vi "Register Check Running.vi"(8 "error in (no error)":errorcluster, 11 "Check Running (F)":bool) -> (0 "error out":errorcluster, 3 "Running?":bool)   [LabVIEW 2013, in "Caraya.lvlib" / "Basic Test Manager.lvclass"]
uses:
  Basic Test Manager.lvclass
  <userlib>/_OpenG.lib/array/array.llb/Conditional Auto-Indexing Tunnel (Variant)__ogtk.vi
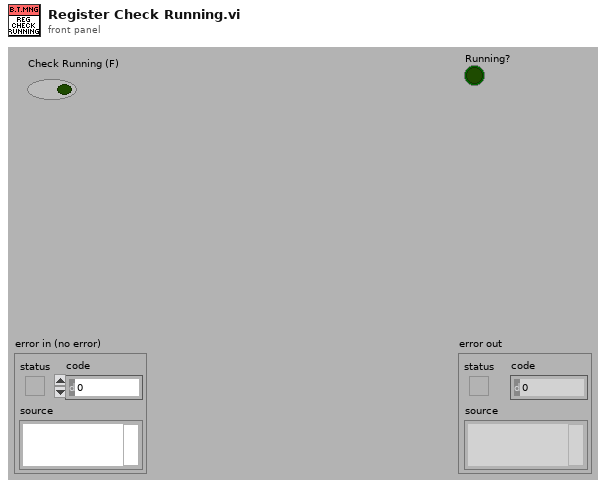
[diagram p1: front panel]
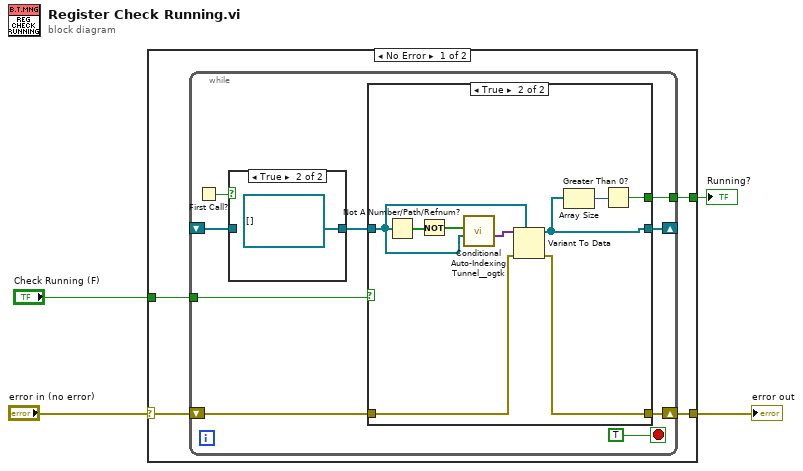
[diagram p0: block diagram]
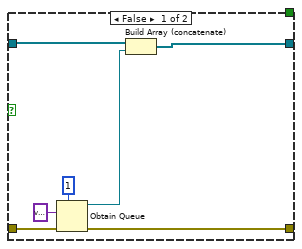
[diagram p3: hidden frame]
diagram:
  n1 = case shown="No Error" "error in (no error)" {
    selector: "error in (no error)" -> [w8 w36]
    tunnel: [w7 w36] -> w3
    tunnel: "Check Running (F)" -> [w6 _]
    tunnel: [w5 _] -> w1
    frame No Error {
      n2 = while {
        shift-right: [w10] -> _
        shift-left: _ -> [w15]
        shift-right: [w11] -> w7
        shift-left: w8 -> [w13]
        tunnel: w6 -> [w12]
        tunnel: [w9] -> w5
        stop <- TRUE stop-if-true
        n3 = First Call?() -> (First Call?: T/F=w16:bool)
        n4 = case shown="True" w16 {
          tunnel: w15 -> [w18 _]
          tunnel: [w18 refnum<queue>[] [] ("Array")] -> w14
          frame False {
          }
          frame True {
          }
        }
        n5 = case shown="True" w12 {
          tunnel: w14 -> [w22 w32]
          tunnel: w13 -> [w26 w31]
          tunnel: [w24 w30] -> w11
          tunnel: [w20 w29] -> w10
          tunnel: [_ w27] -> w9
          frame False {
            n6 = Obtain Queue(max queue size (-1, unlimited)=1, element data type=variant, error in (no error)=w26) -> (queue out=w21:refnum<queue>, error out=w24:errorcluster)  [unwired: 2 in, 1 out]
            n7 = Build Array (concatenate)(w22, w21) -> (w20:refnum<queue>[])
          }
          frame True {
            n8 = Not A Number/Path/Refnum?(number/path/refnum=w32) -> (NaN/Path/Refnum?=w35:bool[])
            n9 = Not(x=w35) -> (.not. x?=w34:bool[])
            n10 = call-poly <userlib>:"Conditional Auto-Indexing Tunnel__ogtk.vi"("Array in"=w32, "Elements to keep"=w34) -> ("Filtered Array out"=w33:variant[])  [unwired: 5 in]
            n11 = Variant To Data(error in=w31, type=w32, Variant=w33) -> (data=w29:refnum<queue>[], error out=w30:errorcluster)
            n12 = Array Size(array=w29) -> (size(s)=w28:i32)
            n13 = Greater Than 0?(x=w28) -> (x > 0?=w27:bool)
          }
        }
      }
    }
    frame Error {
    }
  }
  "error out" <- w3
  "Running?" <- w1
